vi "img.Rotate.vi"(6 "rotate":bool, 9 "image in":u16[][](array[numeric])) -> (1 "image out":u16[][](array[numeric]))   [LabVIEW 2020]
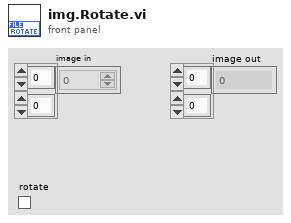
[diagram p1: front panel]
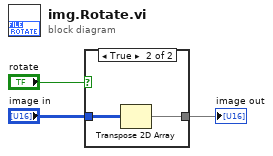
[diagram p0: block diagram]
diagram:
  n1 = case shown="True" "rotate" {
    tunnel: "image in" -> [w4 w6]
    tunnel: [w4 w5] -> w2
    frame False {
    }
    frame True {
      n2 = Transpose 2D Array(2D array=w6) -> (transposed array=w5:u16[][])
    }
  }
  "image out" <- w2
